vi "Subscription Loop.vi"(8 "Init Promise":refnum<class "Promise.lvclass">, 9 "Subscription Info":T1, 10 "Subscription":T2, 11 "ChannelService":refnum<class "ChannelService.lvclass">) -> ()   [LabVIEW 2020, in "Vecto.lvlib" / "RemoteDataService.lvclass"]
uses:
  RemoteDataService.lvclass
  ChannelService/ChannelService.lvclass
  Subscription.ctl
  Subscription Info.ctl
  lv-promises/Promises/Promise/Promise.lvclass
  Subscription State.ctl
  Subscription Loop Data.ctl
  Subscription Group Info.ctl
  GroupAbstract/GroupAbstract.lvclass
  lv-promises/Promises/Error Result/Error Result.lvclass/Error Result.ctl
  lv-promises/Promises/Error Result/Error Result.lvclass
  C:/dev/lv20CE/relink/lv-promises/Promises/Value/Value.lvclass
  <vilib>/Utility/tcp.llb/UDP Multicast Read-Only Open.vi
  <vilib>/Utility/error.llb/Error Cluster From Error Code.vi
  Vecto.lvlib
  proto/GroupData/GroupData.lvlib
  proto/StringData/StringData.lvlib
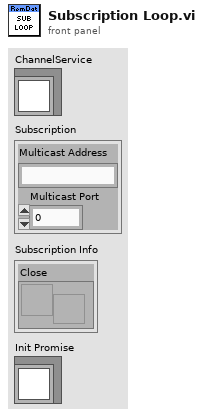
[diagram p1: front panel]
types:
  T1 = typedef "Vecto.lvlib/RemoteDataService.lvclass/Subscription Info.ctl" = cluster{"Close":refnum<user-event>}
  T2 = typedef "Vecto.lvlib/RemoteDataService.lvclass/Subscription.ctl" = cluster{"Multicast Address":string, "Multicast Port":u16}
  T3 = typedef "Vecto.lvlib/RemoteDataService.lvclass/Subscription State.ctl" = enum16{"Init", "Run", "Close"}
  T4 = typedef "Vecto.lvlib/RemoteDataService.lvclass/Subscription Loop Data.ctl" = cluster{"Groups":map{string, T5}}
  T5 = typedef "Vecto.lvlib/RemoteDataService.lvclass/Subscription Group Info.ctl" = cluster{"Last Sequence":u32, "Group":refnum<class "GroupAbstract.lvclass">}
  T6 = typedef "UdpPayload.lvlib/Data.ctl" = cluster{"source_id":u32, "sequence":u32, "timestamp":u64, "type":string, "payload":u8[]}
  T7 = typedef "Vecto.lvlib/Group Data Type.ctl" = enum16{"Double", "String"}
  T8 = typedef "GroupData.lvlib/Data.ctl" = cluster{"group_name":string, "data_timestamp":i64, "scaled_data":dbl[], "raw_data":dbl[]}
  T9 = typedef "StringData.lvlib/Data.ctl" = cluster{"group_name":string, "data_timestamp":i64, "strings":string[]}
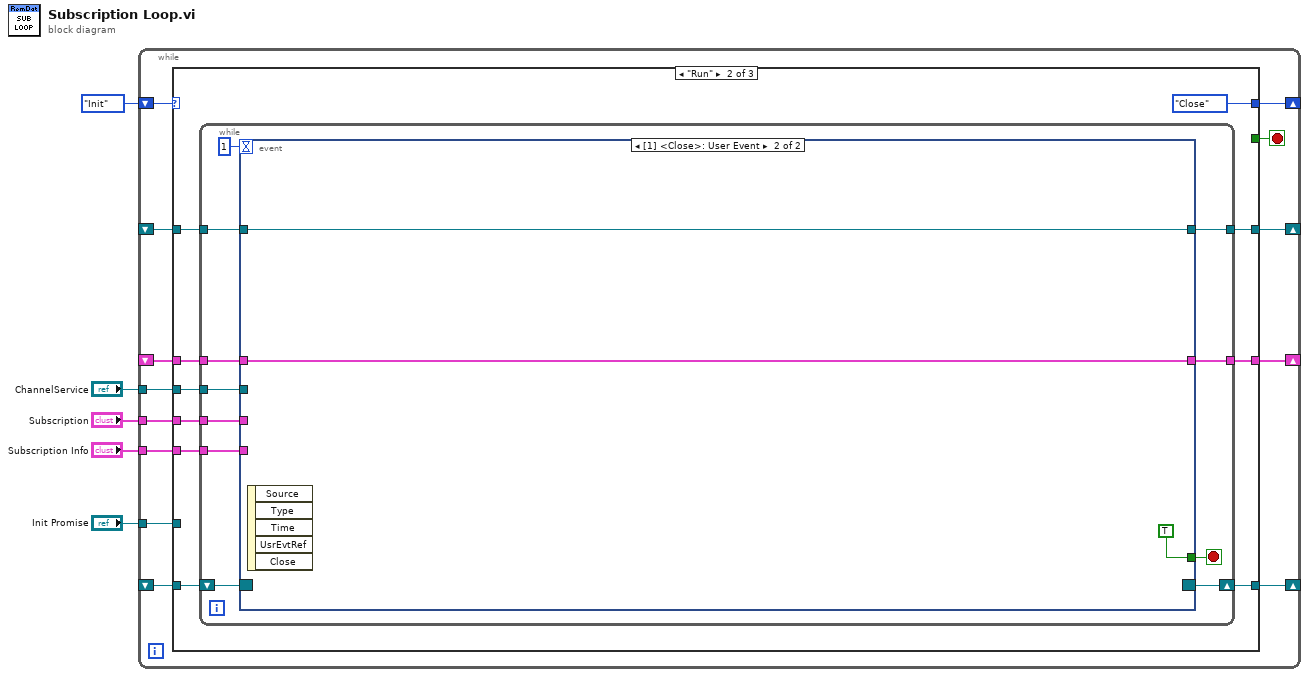
[diagram p0: block diagram]
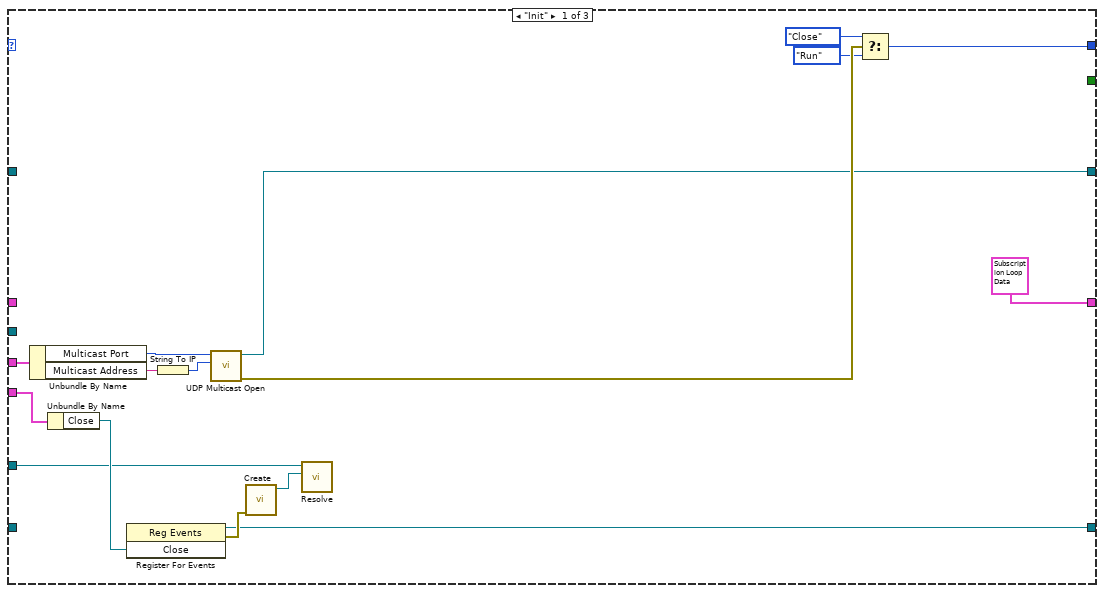
[diagram p2: hidden frame]
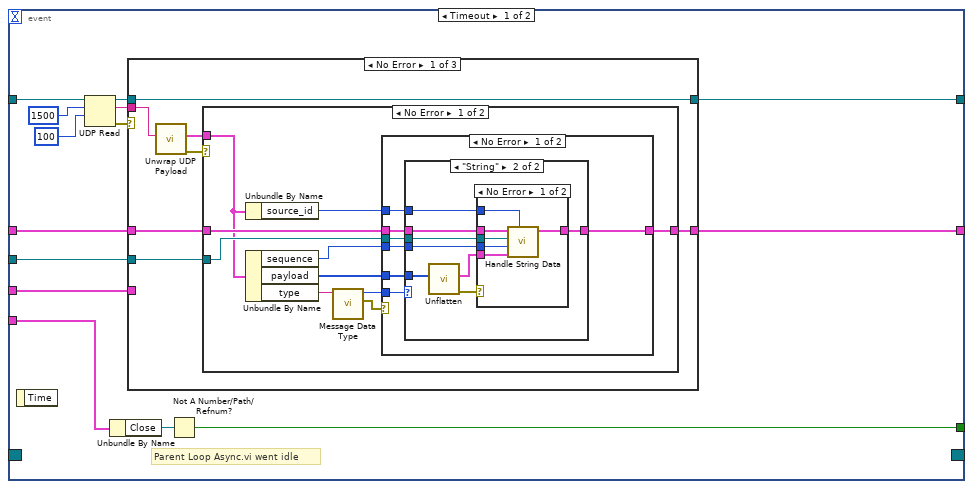
[diagram p3: hidden frame]
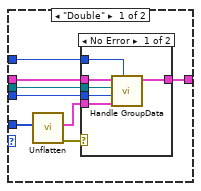
[diagram p4: hidden frame]
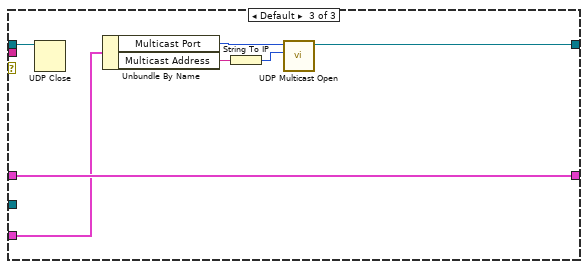
[diagram p10: hidden frame]
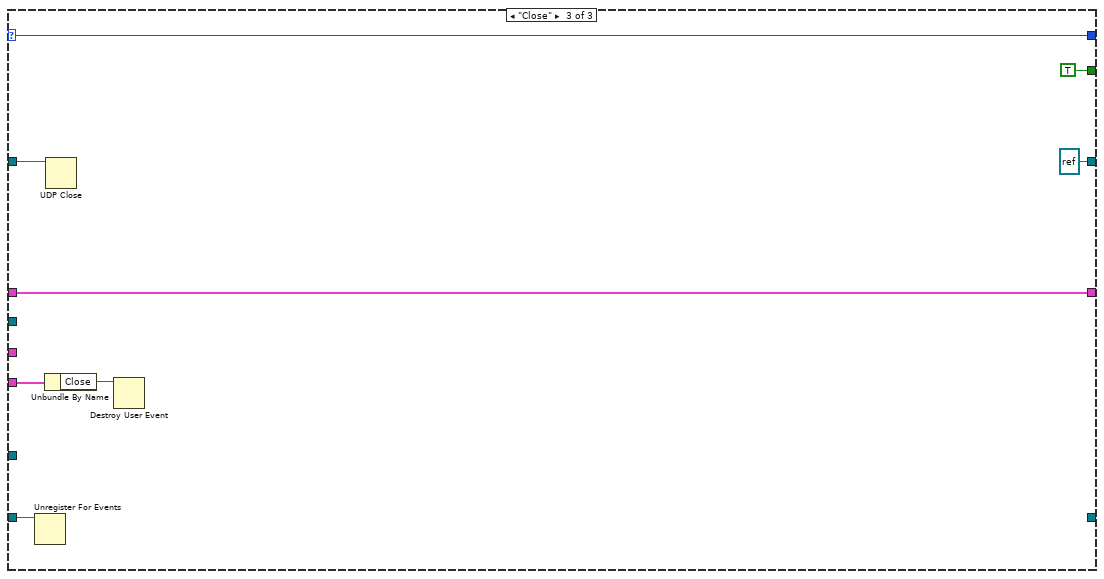
[diagram p11: hidden frame]
diagram:
  n1 = while {
    shift-right: [w17] -> _
    shift-left: Subscription_State."Init" ("Subscription State") -> [w18]
    tunnel: "ChannelService" -> [w16]
    tunnel: "Subscription" -> [w15]
    tunnel: "Subscription Info" -> [w14]
    shift-right: [w12] -> _
    shift-left: _ -> [w11]
    shift-right: [w9] -> _
    shift-left: _ -> [w8]
    shift-right: [w7] -> _
    shift-left: _ -> [w13]
    tunnel: "Init Promise" -> [w6]
    stop <- w10 stop-if-true
    n2 = case shown="\"Run\"" w18 {
      selector: w18 -> [_ _ w145]
      tunnel: [w30 Subscription_State."Close" ("Subscription State") w145] -> w17
      tunnel: w16 -> [_ w42 _]
      tunnel: w15 -> [w29 w39 _]
      tunnel: w14 -> [w23 w38 w144]
      tunnel: w13 -> [_ w43 w142]
      tunnel: [w25 w40 refnum<k16> refnum ("connection ID")] -> w12
      tunnel: w11 -> [_ w41 w141]
      tunnel: [_ _ TRUE] -> w10
      tunnel: [T4 {"Groups"={}} ("Subscription Loop Data") w36 w138] -> w9
      tunnel: w8 -> [_ w37 w138]
      tunnel: [w21 w35 _] -> w7
      tunnel: w6 -> [w20 _ _]
      frame "Init" {
        n3 = Unbundle By Name(w29) -> ("Multicast Port"=w26:u16, "Multicast Address"=w28:string)
        n4 = Unbundle By Name(w23) -> ("Close"=w22:refnum<user-event>)
        n5 = register-events(w22) -> (reference out=w21:refnum<event-registration>, error out=w34:errorcluster)  [unwired: 2 in]
        n6 = String To IP(1:w28) -> (0:w27:u32)
        n7 = call-poly <vilib>:"UDP Multicast Open.vi"("multicast addr"=w27, "port"=w26) -> ("error out"=w33:errorcluster, "connection ID"=w25:refnum<k16>)  [unwired: 7 in, 1 out]
        n8 = call "Create.vi"("error in (no error)"=w34) -> ("Error Result out"=w19:refnum<class "Error Result.lvclass">)  [unwired: 9 in, 1 out]
        n9 = call "Resolve.vi"("Result"=w19, "Promise in"=w20) -> ()  [unwired: 8 in, 2 out]
        n10 = Select(t=Subscription_State."Close" ("Subscription State"), s=w33, f=Subscription_State."Run" ("Subscription State")) -> (s? t:f=w30:T3)
      }
      frame "Run" {
        n11 = while {
          shift-right: [w53] -> w35
          shift-left: w43 -> [w54]
          tunnel: w42 -> [w51]
          tunnel: w41 -> [w50]
          tunnel: [w49] -> w40
          tunnel: w39 -> [w48]
          tunnel: w38 -> [w47]
          tunnel: w37 -> [w46]
          tunnel: [w45] -> w36
          stop <- w52 stop-if-true
          n12 = event shown="[1] <Close>: User Event" {
            selector: w54 -> [_ _]
            dyn-events: [_ _] -> w53
            timeout: 1 -> [_ _]
            tunnel: [w56 TRUE] -> w52
            tunnel: w51 -> [w59 _]
            tunnel: w50 -> [w69 w136]
            tunnel: [w62 w136] -> w49
            tunnel: w48 -> [w60 _]
            tunnel: w47 -> [w58 _]
            tunnel: w46 -> [w63 w135]
            tunnel: [w61 w135] -> w45
            event Timeout {
              # "Parent Loop Async.vi went idle"
              n13 = event-data() -> ()  [unwired: 1 in, 1 out]
              n14 = UDP Read(connection ID=w69, max size (548)=1500, timeout ms (25000)=100) -> (data out=w65:string, error out=w64:errorcluster, 3:w66:refnum<k16>)  [unwired: 1 in, 2 out]
              n15 = Unbundle By Name(w58) -> ("Close"=w57:refnum<user-event>)
              n16 = case shown="No Error" w64 {
                tunnel: w66 -> [w76 w127 w133]
                tunnel: w65 -> [w75 _ _]
                tunnel: w63 -> [w73 w126 w134]
                tunnel: [w76 w127 w129] -> w62
                tunnel: [w70 w126 w134] -> w61
                tunnel: w60 -> [_ _ w128]
                tunnel: w59 -> [w71 _ _]
                frame No Error {
                  n17 = call "Unwrap UDP Payload.vi"("UDP Payload"=w75) -> ("error out"=w74:errorcluster, "Data"=w72:T6)  [unwired: 9 in]
                  n18 = case shown="No Error" w74 {
                    tunnel: w73 -> [w85 w125]
                    tunnel: w72 -> [w81 _]
                    tunnel: w71 -> [w84 _]
                    tunnel: [w82 w125] -> w70
                    frame No Error {
                      n19 = Unbundle By Name(w81) -> ("source_id"=w80:u32)
                      n20 = Unbundle By Name(w81) -> ("sequence"=w83:u32, "payload"=w86:u8[], "type"=w79:string)
                      n21 = call "Message Data Type.vi"("Message Type"=w79) -> ("error out"=w78:errorcluster, "Group Data Type"=w77:T7)  [unwired: 9 in]
                      n22 = case shown="No Error" w78 {
                        tunnel: w86 -> [w93 _]
                        tunnel: w85 -> [w92 w124]
                        tunnel: w84 -> [w91 _]
                        tunnel: w83 -> [w90 _]
                        tunnel: [w89 w124] -> w82
                        tunnel: w80 -> [w88 _]
                        tunnel: w77 -> [w87 _]
                        frame No Error {
                          n23 = case shown="\"String\"" w87 {
                            tunnel: w93 -> [w101 w116]
                            tunnel: w92 -> [w100 w115]
                            tunnel: w91 -> [w99 w114]
                            tunnel: w90 -> [w98 w113]
                            tunnel: [w95 w110] -> w89
                            tunnel: w88 -> [w94 w109]
                            frame "Double" {
                              n24 = call "Unflatten.vi"("Buffer"=w101) -> ("error out"=w96:errorcluster, "Data"=w97:T8)  [unwired: 9 in]
                              n25 = case shown="No Error" w96 {
                                tunnel: w100 -> [w107 w108]
                                tunnel: w99 -> [w106 _]
                                tunnel: w98 -> [w105 _]
                                tunnel: w97 -> [w104 _]
                                tunnel: [w103 w108] -> w95
                                tunnel: w94 -> [w102 _]
                                frame No Error {
                                n26 = call "Handle GroupData.vi"("Source ID"=w102, "GroupData"=w104, "Sequence"=w105, "ChannelService"=w106, "Subscription Loop Data in"=w107) -> ("Subscription Loop Data"=w103:T4)  [unwired: 5 in, 1 out]
                                }
                                frame Error {
                                }
                              }
                            }
                            frame "String" {
                              n27 = call "Unflatten.vi"("Buffer"=w116) -> ("error out"=w111:errorcluster, "Data"=w112:T9)  [unwired: 9 in]
                              n28 = case shown="No Error" w111 {
                                tunnel: w115 -> [w122 w123]
                                tunnel: w114 -> [w121 _]
                                tunnel: w113 -> [w120 _]
                                tunnel: w112 -> [w119 _]
                                tunnel: [w118 w123] -> w110
                                tunnel: w109 -> [w117 _]
                                frame No Error {
                                n29 = call "Handle String Data.vi"("Source ID"=w117, "StringData"=w119, "Sequence"=w120, "ChannelService"=w121, "Subscription Loop Data in"=w122) -> ("Subscription Loop Data"=w118:T4)  [unwired: 5 in, 1 out]
                                }
                                frame Error {
                                }
                              }
                            }
                          }
                        }
                        frame Error {
                        }
                      }
                    }
                    frame Error {
                    }
                  }
                }
                frame Error {
                }
                frame Default {
                  n30 = UDP Close(connection ID=w133) -> ()  [unwired: 1 in, 2 out]
                  n31 = Unbundle By Name(w128) -> ("Multicast Port"=w130:u16, "Multicast Address"=w132:string)
                  n32 = String To IP(1:w132) -> (0:w131:u32)
                  n33 = call-poly <vilib>:"UDP Multicast Open.vi"("multicast addr"=w131, "port"=w130) -> ("connection ID"=w129:refnum<k16>)  [unwired: 7 in, 2 out]
                }
              }
              n34 = Not A Number/Path/Refnum?(number/path/refnum=w57) -> (NaN/Path/Refnum?=w56:bool)
            }
            event User Event {
              n35 = event-data() -> ()  [unwired: 1 in, 5 out]
            }
          }
        }
      }
      frame "Close" {
        n36 = Unregister For Events(event registration refnum=w142) -> ()  [unwired: 1 in, 1 out]
        n37 = Unbundle By Name(w144) -> ("Close"=w143:refnum<user-event>)
        n38 = UDP Close(connection ID=w141) -> ()  [unwired: 1 in, 2 out]
        n39 = Destroy User Event(user event=w143) -> ()  [unwired: 1 in, 1 out]
      }
    }
  }
